vi "menuItemsWorkaround_send.vi"(11 "flatMenu[]":T1) -> ()   [LabVIEW 2013]
uses:
  flatMenu.ctl
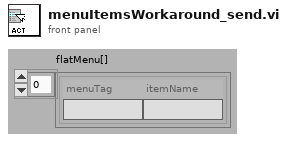
[diagram p1: front panel]
types:
  T1 = typedef "flatMenu.ctl" = cluster{"menuTag":string, "itemName":string}[]
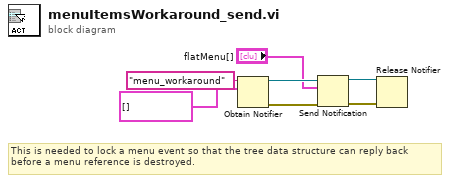
[diagram p0: block diagram]
diagram:
  # "This is needed to lock a menu event so that the tree data structure can reply back \nbefore a menu reference is destroyed."
  n1 = Obtain Notifier(name (unnamed)="menu_workaround", notification data type=T1 [] ("flatMenu[]")) -> (notifier out=w5:refnum<notifier>, error out=w6:errorcluster)  [unwired: 2 in, 1 out]
  n2 = Send Notification(notification="flatMenu[]", notifier=w5, error in (no error)=w6) -> (notifier out=w7:refnum<notifier>, error out=w3:errorcluster)
  n3 = Release Notifier(notifier=w7, error in (no error)=w3) -> ()  [unwired: 1 in, 3 out]
